vi "Example 5 - RMX410x Configuration.vi"(8 "error in (no error)":errorcluster) -> (0 "error out":errorcluster)   [LabVIEW 2018]
uses:
  <vilib>/addons/VeriStand Custom Device Scripting APIs/Instrument Addon/Libraries Directory/Protocols.lvlibp/RS-xxx/RS-xxx Settings.ctl
  <vilib>/addons/VeriStand Custom Device Scripting APIs/Instrument Addon/API/TypeDefs/Message Settings.ctl
  <vilib>/addons/VeriStand Custom Device Scripting APIs/Instrument Addon/API/TypeDefs/Protection Types.ctl
  <vilib>/addons/VeriStand Custom Device Scripting APIs/Instrument Addon/API/TypeDefs/Single Channel Enumerated List Settings.ctl
  <vilib>/NI Veristand/Custom Device API/Custom Device Item Ref.ctl
  <vilib>/addons/VeriStand Custom Device Scripting APIs/Instrument Addon/API/TypeDefs/Command Settings.ctl
  <vilib>/addons/VeriStand Custom Device Scripting APIs/Instrument Addon/API/TypeDefs/Padding.ctl
  <vilib>/addons/VeriStand Custom Device Scripting APIs/Instrument Addon/API/TypeDefs/ByteCount Response Settings.ctl
  <vilib>/addons/VeriStand Custom Device Scripting APIs/Instrument Addon/API/TypeDefs/Linked Channel.ctl
  <vilib>/addons/VeriStand Custom Device Scripting APIs/Instrument Addon/API/TypeDefs/Single Channel Format Settings.ctl
  NationalInstruments.VeriStand.SystemDefinitionAPI
  <vilib>/addons/VeriStand Custom Device Scripting APIs/Instrument Addon/API/Custom Device/RS-xxx Factory.vi
  <vilib>/addons/VeriStand Custom Device Scripting APIs/Instrument Addon/API/Messages/Create Message - Periodic & Trigger.vi
  <vilib>/addons/VeriStand Custom Device Scripting APIs/Instrument Addon/API/Channels/Create Data Channel - Single Channel - Format.vi
  <vilib>/addons/VeriStand Custom Device Scripting APIs/Instrument Addon/API/Messages/Configure Response - Byte Count.vi
  <vilib>/addons/VeriStand Custom Device Scripting APIs/Instrument Addon/API/Channels/Create Data Channel - Single Channel - Enumerated List.vi
  <vilib>/addons/VeriStand Custom Device Scripting APIs/Instrument Addon/API/Messages/Create Message - Value Change & Trigger.vi
  <vilib>/addons/VeriStand Custom Device Scripting APIs/Instrument Addon/API/Channels/Create MetaData Channel - Single Channel - Format.vi
  <vilib>/addons/VeriStand Custom Device Scripting APIs/Instrument Addon/API/Channels/Create MetaData Channel - Single Channel - Enumerated List.vi
  <vilib>/addons/VeriStand Custom Device Scripting APIs/Instrument Addon/API/Instrument Addon Scripting API.lvlib
  <vilib>/addons/VeriStand Custom Device Scripting APIs/Instrument Addon/Libraries Directory/Protocols.lvlibp/RS-xxx/RS-xxx.lvclass
  <vilib>/NI Veristand/Custom Device API/Custom Device API.lvlib
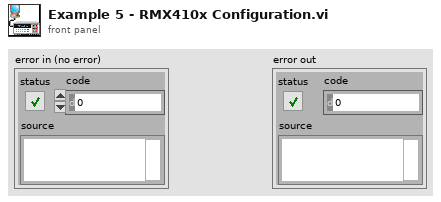
[diagram p1: front panel]
types:
  T1 = typedef "Instrument Addon Scripting API.lvlib/Linked Channel.ctl" = cluster{"Variable Name":string, "Channel Refnum":T2}
  T2 = typedef "Custom Device API.lvlib/Custom Device Item Ref.ctl" = u64
  T3 = typedef "Instrument Addon Scripting API.lvlib/ByteCount Response Settings.ctl" = cluster{"Response Format":string, "Linked Channels":T1[], "Byte Count":i32, "Use Byte Count channel":bool, "Channel Refnum":T2}
  T4 = typedef "Instrument Addon Scripting API.lvlib/Single Channel Format Settings.ctl" = cluster{"Format String":string, "Default Value":dbl, "Units":string}
  T5 = typedef "Instrument Addon Scripting API.lvlib/Single Channel Enumerated List Settings.ctl" = cluster{"Enumerated List":string[], "Default Value":dbl, "Units":string}
  T6 = cluster{"Variable Name":string, "Channel Ref in":T2}
  T7 = typedef "Instrument Addon Scripting API.lvlib/Command Settings.ctl" = cluster{"Command Format":string, "Linked Channels":cluster{"Variable Name":string, "Channel Ref in":T2}[], "Use Padding?":bool, "Padding":T8}
  T8 = typedef "Instrument Addon Scripting API.lvlib/Padding.ctl" = cluster{"Pad Value":u8, "Length":u32}
  T9 = typedef "Instrument Addon Scripting API.lvlib/Protection Types.ctl" = enum16{"None", "CRC-32", "Checksum U16", "Checksum U32", "Checksum U8"}
  T10 = typedef "Instrument Addon Scripting API.lvlib/Message Settings.ctl" = cluster{"Protection":T9, "Enable Periodic Default":bool, "Trigger Channel refnum":u64}
  T11 = enum16{"NUL", "SOH", "STX", "ETX", "EOT", "ENQ", "ACK", "BEL", "BS", "HT", "LF", "VT", "FF", "CR", "SO", "SI", "DLE", "DC1", "DC2", "DC3", "DC4", "NAK", "SYN", "ETB", "CAN", "EM", "SUB", "ESC", "FS", "GS", "RS", "US", "SP", "!", "\"", "#", "$", "%", "&", "'", "(", ")", "*", "+", ",", "- (-)", ".", "/", "0", "1", "2", "3", "4", "5", "6", "7", "8", "9", ":", ";", "<", "=", ">", "?", "@", "A", "B", "C", "D", "E", "F", "G", "H", "I", "J", "K", "L", "M", "N", "O", "P", "Q", "R", "S", "T", "U", "V", "W", "X", "Y", "Z", "[", "\\", "]", "^", "_", "`", "a", "b", "c", "d", "e", "f", "g", "h", "i", "j", "k", "l", "m", "n", "o", "p", "q", "r", "s", "t", "u", "v", "w", "x", "y", "z", "{", "|", "}", "~"}
  T12 = typedef "Protocols.lvlibp/RS-xxx.lvclass/RS-xxx Settings.ctl" = cluster{"Port":string, "Baud Rate":u32, "Data Bits":u16, "Parity":enum16{"None", "Odd", "Even", "Mark", "Space"}, "Stop Bits":u16, "Flow Control":u16, "XON":enum16{"NUL", "SOH", "STX", "ETX", "EOT", "ENQ", "ACK", "BEL", "BS", "HT", "LF", "VT", "FF", "CR", "SO", "SI", "DLE", "DC1", "DC2", "DC3", "DC4", "NAK", "SYN", "ETB", "CAN", "EM", "SUB", "ESC", "FS", "GS", "RS", "US", "SP", "!", "\"", "#", "$", "%", "&", "'", "(", ")", "*", "+", ",", "- (-)", ".", "/", "0", "1", "2", "3", "4", "5", "6", "7", "8", "9", ":", ";", "<", "=", ">", "?", "@", "A", "B", "C", "D", "E", "F", "G", "H", "I", "J", "K", "L", "M", "N", "O", "P", "Q", "R", "S", "T", "U", "V", "W", "X", "Y", "Z", "[", "\\", "]", "^", "_", "`", "a", "b", "c", "d", "e", "f", "g", "h", "i", "j", "k", "l", "m", "n", "o", "p", "q", "r", "s", "t", "u", "v", "w", "x", "y", "z", "{", "|", "}", "~"}, "XOFF":enum16{"NUL", "SOH", "STX", "ETX", "EOT", "ENQ", "ACK", "BEL", "BS", "HT", "LF", "VT", "FF", "CR", "SO", "SI", "DLE", "DC1", "DC2", "DC3", "DC4", "NAK", "SYN", "ETB", "CAN", "EM", "SUB", "ESC", "FS", "GS", "RS", "US", "SP", "!", "\"", "#", "$", "%", "&", "'", "(", ")", "*", "+", ",", "- (-)", ".", "/", "0", "1", "2", "3", "4", "5", "6", "7", "8", "9", ":", ";", "<", "=", ">", "?", "@", "A", "B", "C", "D", "E", "F", "G", "H", "I", "J", "K", "L", "M", "N", "O", "P", "Q", "R", "S", "T", "U", "V", "W", "X", "Y", "Z", "[", "\\", "]", "^", "_", "`", "a", "b", "c", "d", "e", "f", "g", "h", "i", "j", "k", "l", "m", "n", "o", "p", "q", "r", "s", "t", "u", "v", "w", "x", "y", "z", "{", "|", "}", "~"}, "End Read on Termination Character":bool, "End Write on Termination Character":bool, "Termination Character":u8}
  T13 = cluster{"Variable Name":string, "Channel Ref in":T2}[]
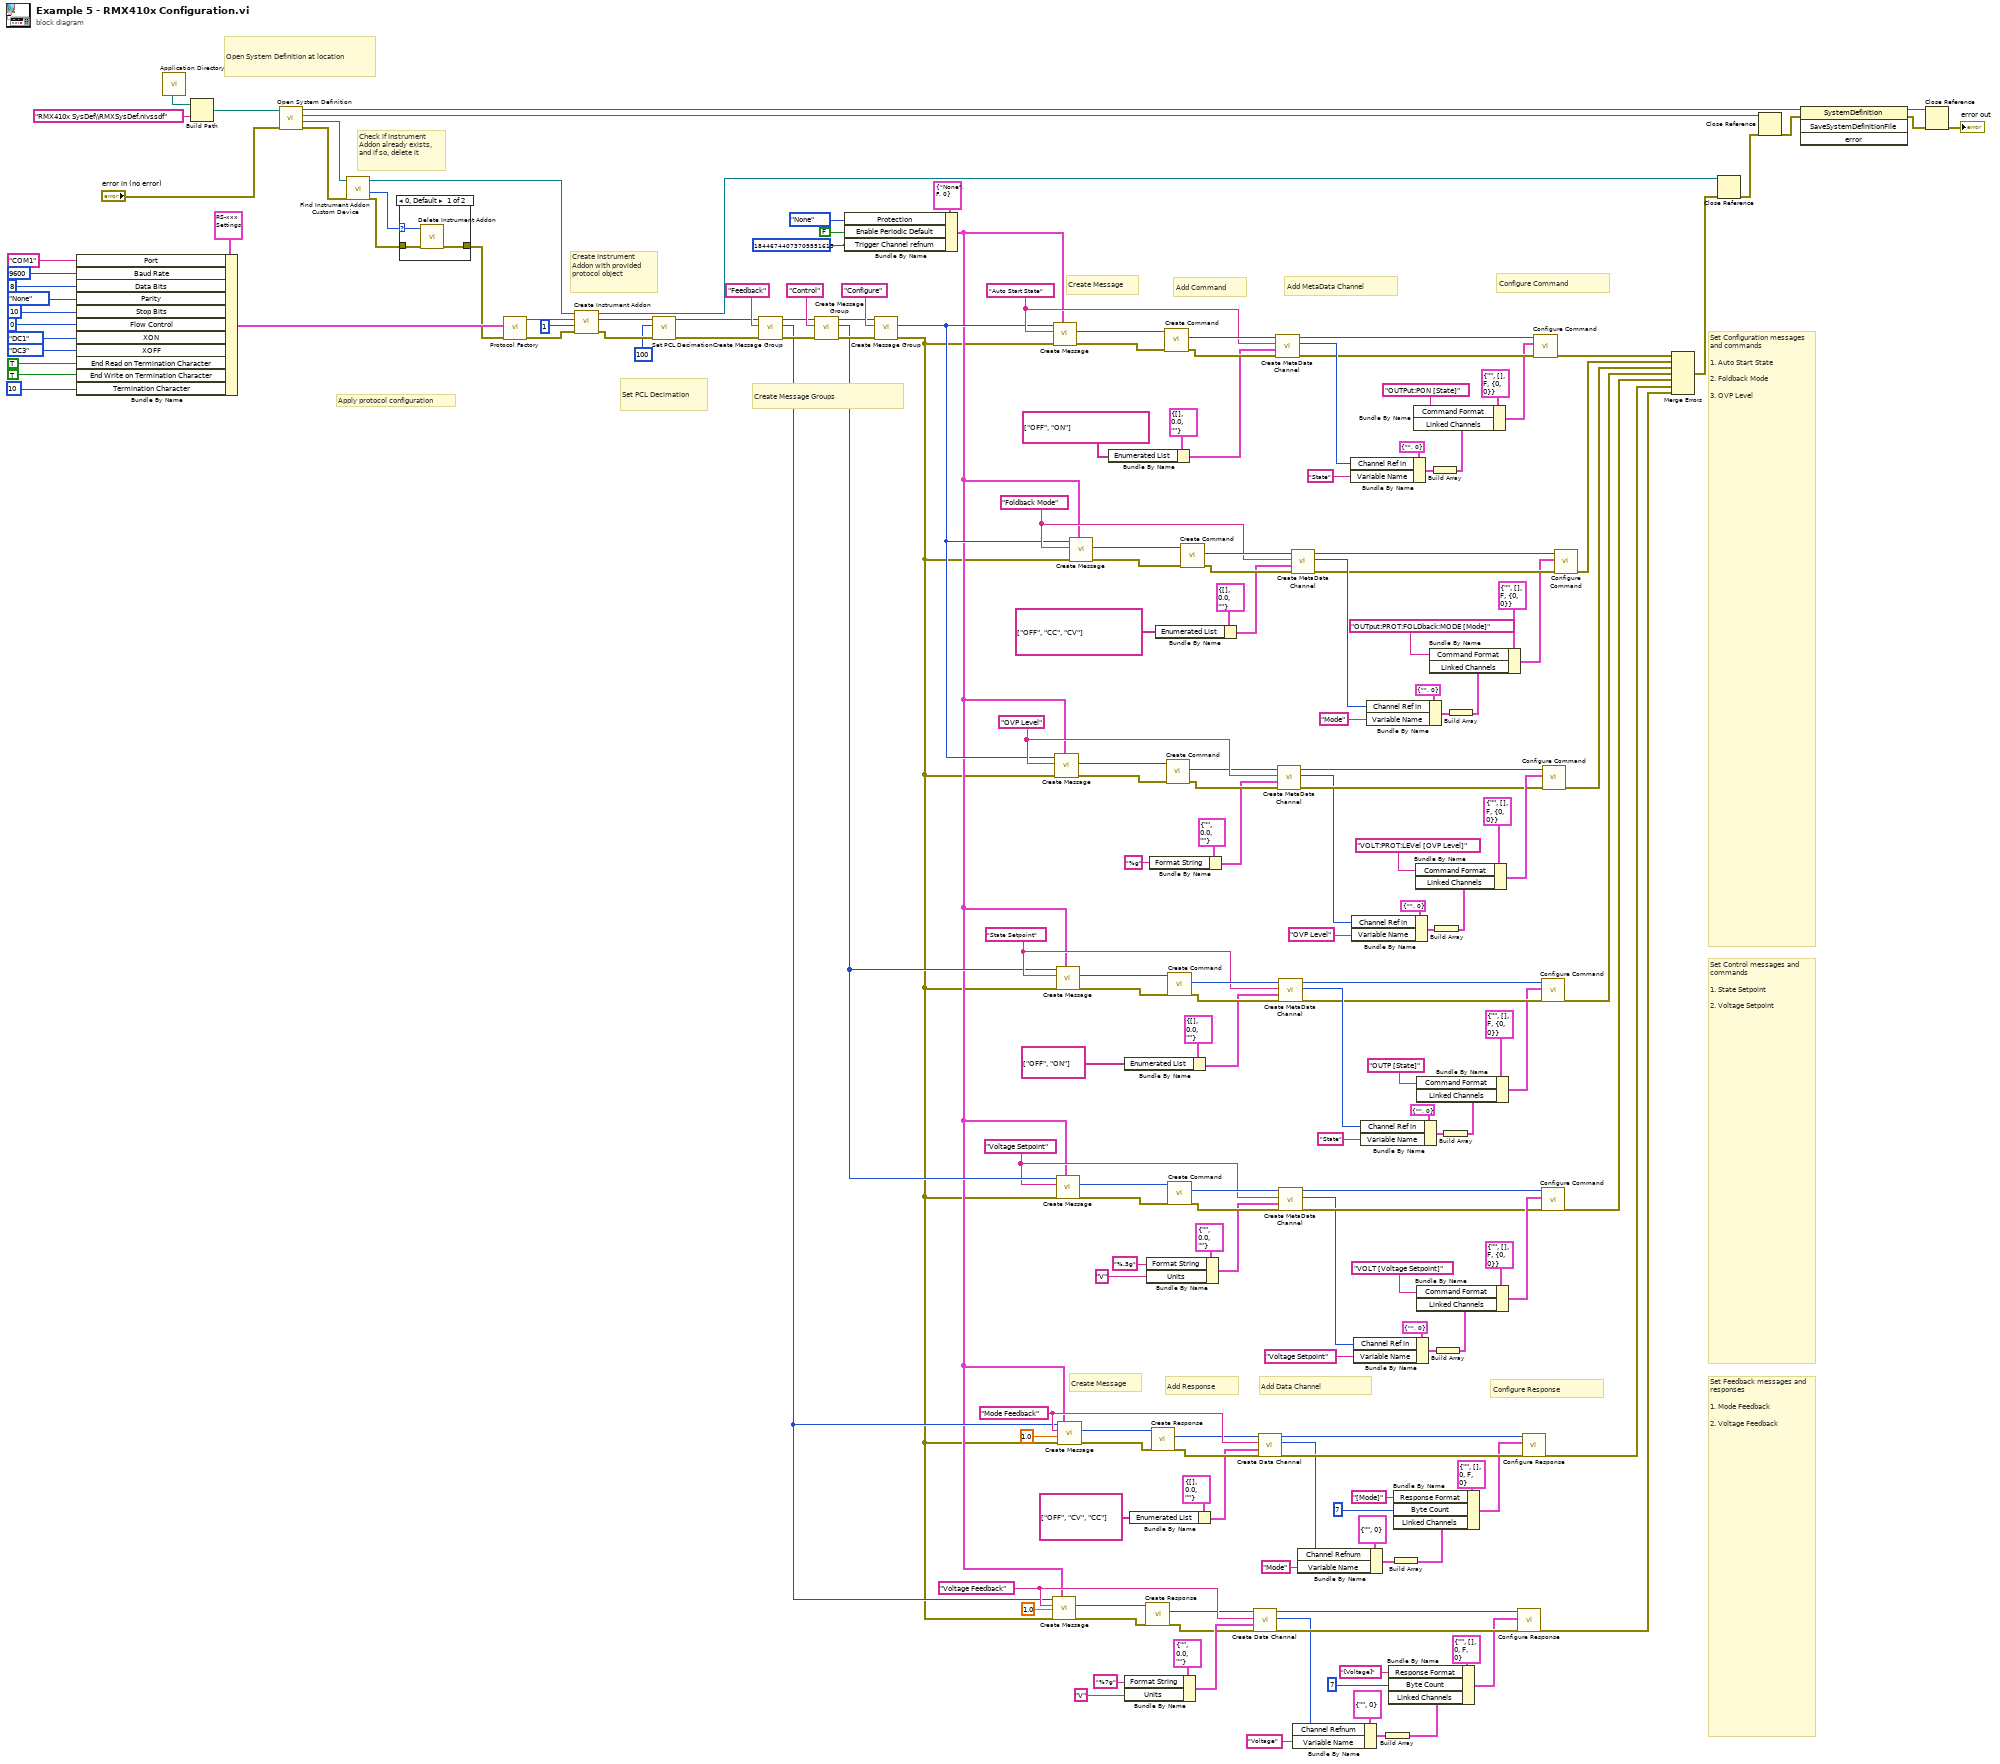
[diagram p0: block diagram]
diagram:
  w17 = "Voltage Feedback" ("message name")
  w40 = "Mode Feedback" ("message name")
  w58 = "Voltage Setpoint" ("message name")
  w78 = "State Setpoint" ("message name")
  w117 = "OVP Level" ("message name")
  w120 = "Foldback Mode" ("message name")
  w119 = "Auto Start State" ("message name")
  # "Create Instrument Addon with provided protocol object"
  # "Open System Definition at location"
  # "Configure Response"
  # "Add Data Channel"
  # "Add Response"
  # "Create Message"
  # "Configure Command"
  # "Add MetaData Channel"
  # "Add Command"
  # "Create Message"
  # "Set Feedback messages and responses\n\n1. Mode Feedback\n\n2. Voltage Feedback"
  # "Set Control messages and commands\n\n1. State Setpoint\n\n2. Voltage Setpoint"
  # "Set Configuration messages and commands\n\n1. Auto Start State\n\n2. Foldback Mode\n\n3. OVP Level"
  # "Create Message Groups"
  # "Set PCL Decimation"
  # "Check if Instrument Addon already exists, and if so, delete it"
  # "Apply protocol configuration"
  n1 = Bundle By Name(cluster=T12 {"Port"="", "Baud Rate"=0, "Data Bits"=0, "Parity"=enum."None", "Stop Bits"=0, "Flow Control"=0, "XON"=enum."NUL", "XOFF"=enum."NUL", "End Read on Termination Character"=FALSE, "End Write on Termination Character"=FALSE, "Termination Character"=0} ("RS-xxx settings"), "Port"="COM1", "Baud Rate"=u32 9600, "Data Bits"=u16 8, "Parity"=enum16{"None", "Odd", "Even", "Mark", "Space"}."None", "Stop Bits"=u16 10, "Flow Control"=u16 0, "XON"=T11."DC1", "XOFF"=T11."DC3", "End Read on Termination Character"=TRUE, "End Write on Termination Character"=TRUE ("End Read on Termination Character"), "Termination Character"=u8 10) -> (w193:T12)
  n2 = call <vilib>:"Application Directory.vi"() -> ("Application Directory"=w180:path)
  n3 = Build Path(base path=w180, name or relative path="RMX410x SysDef\\RMXSysDef.nivssdf") -> (appended path=w178:path)
  n4 = call "Open System Definition.vi"("error in (no error)"="error in (no error)", "System Definition File"=w178) -> ("error out"=w166:errorcluster, "Target Refnum"=w168:refnum<k24>, "Root Refnum"=w177:refnum<k24>, "System Definition Refnum"=w172:refnum<k24>)  [unwired: 6 in]
  n5 = call "Find Instrument Addon Custom Device.vi"("error in"=w166, "target in"=w168) -> ("error out"=w165:errorcluster, "NodeID"=w147:u64, "target out"=w163:refnum<k24>)  [unwired: 7 in]
  n6 = case shown="0, Default" w147 {
    selector: w147 -> [w196 _]
    tunnel: w165 -> [w198 w199]
    tunnel: [w197 w199] -> w164
    frame 0, Default {
      n7 = call <vilib>:"Delete Instrument Addon.vi"("error in (no error)"=w198, "instrument addon refnum"=w196) -> ("error out"=w197:errorcluster)  [unwired: 9 in]
    }
    frame -1 {
    }
  }
  n8 = call-poly <vilib>:"Protocol Factory.vi"("error in (no error)"=w164, "RS-xxx settings"=w193) -> ("error out"=w175:errorcluster, "protocol out"=w195:refnum<class "Protocol Parent.lvclass">)  [unwired: 8 in]
  n9 = call <vilib>:"Create Instrument Addon.vi"("error in (no error)"=w175, "PCL decimation"=u16 1, "protocol in"=w195, "target in"=w163) -> ("error out"=w8:errorcluster, "instrument addon refnum"=w9:T2, "target out"=w176:refnum<k24>)  [unwired: 5 in]
  n10 = call <vilib>:"Set PCL Decimation.vi"("error in (no error)"=w8, "PCL decimation"=u32 100, "instrument addon refnum in"=w9) -> ("error out"=w6:errorcluster, "instrument addon refnum"=w7:T2)  [unwired: 7 in]
  n11 = call <vilib>:"Create Message Group.vi"("error in (no error)"=w6, "message group name"="Feedback", "instrument addon refnum in"=w7) -> ("error out"=w95:errorcluster, "message group refnum out"=w12:T2, "instrument addon refnum out"=w96:T2)  [unwired: 6 in]
  n12 = call <vilib>:"Create Message Group.vi"("error in (no error)"=w95, "message group name"="Control", "instrument addon refnum in"=w96) -> ("error out"=w93:errorcluster, "message group refnum out"=w59:T2, "instrument addon refnum out"=w94:T2)  [unwired: 6 in]
  n13 = Bundle By Name(cluster=T10 {"Protection"=enum."None", "Enable Periodic Default"=FALSE, "Trigger Channel refnum"=0} ("optional settings"), "Protection"=Protection_Types."None", "Enable Periodic Default"=FALSE, "Trigger Channel refnum"=T2 18446744073709551615 ("command refnum")) -> (w4:T10)
  n14 = call <vilib>:"Create Message Group.vi"("error in (no error)"=w93, "message group name"="Configure", "instrument addon refnum in"=w94) -> ("error out"=w3:errorcluster, "message group refnum out"=w74:T2)  [unwired: 6 in, 1 out]
  n15 = call-poly <vilib>:"Create Message.vi"("optional settings"=w4, "error in (no error)"=w3, "period (s)"=1.0, "message name"=w17, "message group refnum in"=w12) -> ("error out"=w14:errorcluster, "message refnum out"=w13:T2)  [unwired: 4 in, 1 out]
  n16 = call-poly <vilib>:"Create Message.vi"("optional settings"=w4, "error in (no error)"=w3, "message name"=w119, "message group refnum in"=w74) -> ("error out"=w160:errorcluster, "message refnum out"=w161:T2)  [unwired: 5 in, 1 out]
  n17 = call-poly <vilib>:"Create Message.vi"("optional settings"=w4, "error in (no error)"=w3, "message name"=w117, "message group refnum in"=w74) -> ("error out"=w104:errorcluster, "message refnum out"=w103:T2)  [unwired: 5 in, 1 out]
  n18 = call-poly <vilib>:"Create Message.vi"("optional settings"=w4, "error in (no error)"=w3, "message name"=w78, "message group refnum in"=w59) -> ("error out"=w91:errorcluster, "message refnum out"=w92:T2)  [unwired: 5 in, 1 out]
  n19 = call-poly <vilib>:"Create Message.vi"("optional settings"=w4, "error in (no error)"=w3, "message name"=w58, "message group refnum in"=w59) -> ("error out"=w61:errorcluster, "message refnum out"=w60:T2)  [unwired: 5 in, 1 out]
  n20 = call-poly <vilib>:"Create Message.vi"("optional settings"=w4, "error in (no error)"=w3, "period (s)"=1.0, "message name"=w40, "message group refnum in"=w12) -> ("error out"=w37:errorcluster, "message refnum out"=w36:T2)  [unwired: 4 in, 1 out]
  n21 = call-poly <vilib>:"Create Message.vi"("optional settings"=w4, "error in (no error)"=w3, "message name"=w120, "message group refnum in"=w74) -> ("error out"=w136:errorcluster, "message refnum out"=w137:T2)  [unwired: 5 in, 1 out]
  n22 = Bundle By Name(cluster=T5 {"Enumerated List"=[], "Default Value"=0.0, "Units"=""} ("settings"), "Enumerated List"=string[] ["OFF", "ON"]) -> (w155:T5)
  n23 = Bundle By Name(cluster=T5 {"Enumerated List"=[], "Default Value"=0.0, "Units"=""} ("settings"), "Enumerated List"=string[] ["OFF", "ON"]) -> (w76:T5)
  n24 = Bundle By Name(cluster=T4 {"Format String"="", "Default Value"=0.0, "Units"=""} ("settings"), "Format String"="%7g", "Units"="V") -> (w19:T4)
  n25 = Bundle By Name(cluster=T5 {"Enumerated List"=[], "Default Value"=0.0, "Units"=""} ("settings"), "Enumerated List"=string[] ["OFF", "CV", "CC"]) -> (w34:T5)
  n26 = call <vilib>:"Create Response.vi"("error in (no error)"=w14, "message refnum in"=w13) -> ("error out"=w16:errorcluster, "response refnum"=w15:T2)  [unwired: 7 in, 1 out]
  n27 = Bundle By Name(cluster=T4 {"Format String"="", "Default Value"=0.0, "Units"=""} ("settings"), "Format String"="%.3g", "Units"="V") -> (w56:T4)
  n28 = Bundle By Name(cluster=T4 {"Format String"="", "Default Value"=0.0, "Units"=""} ("settings"), "Format String"="%g") -> (w101:T4)
  n29 = call <vilib>:"Create Response.vi"("error in (no error)"=w37, "message refnum in"=w36) -> ("error out"=w39:errorcluster, "response refnum"=w38:T2)  [unwired: 7 in, 1 out]
  n30 = Bundle By Name(cluster=T5 {"Enumerated List"=[], "Default Value"=0.0, "Units"=""} ("settings"), "Enumerated List"=string[] ["OFF", "CC", "CV"]) -> (w131:T5)
  n31 = call <vilib>:"Create Command.vi"("error in"=w160, "message refnum In"=w161) -> ("error out"=w158:errorcluster, "command refnum"=w159:T2)  [unwired: 7 in, 1 out]
  n32 = call <vilib>:"Create Command.vi"("error in"=w104, "message refnum In"=w103) -> ("error out"=w106:errorcluster, "command refnum"=w105:T2)  [unwired: 7 in, 1 out]
  n33 = call <vilib>:"Create Command.vi"("error in"=w91, "message refnum In"=w92) -> ("error out"=w89:errorcluster, "command refnum"=w90:T2)  [unwired: 7 in, 1 out]
  n34 = call <vilib>:"Create Command.vi"("error in"=w61, "message refnum In"=w60) -> ("error out"=w63:errorcluster, "command refnum"=w62:T2)  [unwired: 7 in, 1 out]
  n35 = call <vilib>:"Create Command.vi"("error in"=w136, "message refnum In"=w137) -> ("error out"=w134:errorcluster, "command refnum"=w135:T2)  [unwired: 7 in, 1 out]
  n36 = call-poly <vilib>:"Create Data Channel.vi"("error in (no error)"=w16, "settings"=w19, "channel name"=w17, "response refnum in"=w15) -> ("error out"=w32:errorcluster, "channel refnum"=w27:T2, "response refnum out"=w22:T2)  [unwired: 5 in]
  n37 = call-poly <vilib>:"Create Data Channel.vi"("error in (no error)"=w39, "settings"=w34, "channel name"=w40, "response refnum in"=w38) -> ("error out"=w51:errorcluster, "channel refnum"=w46:T2, "response refnum out"=w41:T2)  [unwired: 5 in]
  n38 = call-poly <vilib>:"Create MetaData Channel.vi"("error in (no error)"=w158, "settings"=w155, "channel name"=w119, "command refnum in"=w159) -> ("error out"=w152:errorcluster, "channel refnum"=w153:T2, "command refnum out"=w154:T2)  [unwired: 5 in]
  n39 = call-poly <vilib>:"Create MetaData Channel.vi"("error in (no error)"=w106, "settings"=w101, "channel name"=w117, "command refnum in"=w105) -> ("error out"=w109:errorcluster, "channel refnum"=w108:T2, "command refnum out"=w107:T2)  [unwired: 5 in]
  n40 = call-poly <vilib>:"Create MetaData Channel.vi"("error in (no error)"=w89, "settings"=w76, "channel name"=w78, "command refnum in"=w90) -> ("error out"=w86:errorcluster, "channel refnum"=w87:T2, "command refnum out"=w88:T2)  [unwired: 5 in]
  n41 = call-poly <vilib>:"Create MetaData Channel.vi"("error in (no error)"=w63, "settings"=w56, "channel name"=w58, "command refnum in"=w62) -> ("error out"=w66:errorcluster, "channel refnum"=w65:T2, "command refnum out"=w64:T2)  [unwired: 5 in]
  n42 = call-poly <vilib>:"Create MetaData Channel.vi"("error in (no error)"=w134, "settings"=w131, "channel name"=w120, "command refnum in"=w135) -> ("error out"=w128:errorcluster, "channel refnum"=w129:T2, "command refnum out"=w130:T2)  [unwired: 5 in]
  n43 = Bundle By Name(cluster=T1 {"Variable Name"="", "Channel Refnum"=0} ("Linked Channel"), "Channel Refnum"=w27, "Variable Name"="Voltage") -> (w29:T1)
  n44 = Bundle By Name(cluster=T1 {"Variable Name"="", "Channel Refnum"=0} ("Linked Channel"), "Channel Refnum"=w46, "Variable Name"="Mode") -> (w48:T1)
  n45 = Bundle By Name(cluster=T6 {"Variable Name"="", "Channel Ref in"=0} ("Linked Channel"), "Channel Ref in"=w153, "Variable Name"="State") -> (w142:T6)
  n46 = Bundle By Name(cluster=T6 {"Variable Name"="", "Channel Ref in"=0} ("Linked Channel"), "Channel Ref in"=w108, "Variable Name"="OVP Level") -> (w114:T6)
  n47 = Bundle By Name(cluster=T6 {"Variable Name"="", "Channel Ref in"=0} ("Linked Channel"), "Channel Ref in"=w65, "Variable Name"="Voltage Setpoint") -> (w71:T6)
  n48 = Bundle By Name(cluster=T6 {"Variable Name"="", "Channel Ref in"=0} ("Linked Channel"), "Channel Ref in"=w87, "Variable Name"="State") -> (w81:T6)
  n49 = Bundle By Name(cluster=T6 {"Variable Name"="", "Channel Ref in"=0} ("Linked Channel"), "Channel Ref in"=w129, "Variable Name"="Mode") -> (w123:T6)
  n50 = Build Array(w29) -> (w30:T1[])
  n51 = Bundle By Name(cluster=T3 {"Response Format"="", "Linked Channels"=[], "Byte Count"=0, "Use Byte Count channel"=FALSE, "Channel Refnum"=0} ("settings"), "Response Format"="[Voltage]", "Byte Count"=7, "Linked Channels"=w30) -> (w25:T3)
  n52 = Build Array(w48) -> (w49:T1[])
  n53 = Bundle By Name(cluster=T3 {"Response Format"="", "Linked Channels"=[], "Byte Count"=0, "Use Byte Count channel"=FALSE, "Channel Refnum"=0} ("settings"), "Response Format"="[Mode]", "Byte Count"=7, "Linked Channels"=w49) -> (w44:T3)
  n54 = Build Array(w142) -> (w141:T13)
  n55 = Bundle By Name(cluster=T7 {"Command Format"="", "Linked Channels"=[], "Use Padding?"=FALSE, "Padding"={"Pad Value"=0, "Length"=0}} ("settings"), "Command Format"="OUTPut:PON [State]", "Linked Channels"=w141) -> (w140:T7)
  n56 = Build Array(w114) -> (w115:T13)
  n57 = Bundle By Name(cluster=T7 {"Command Format"="", "Linked Channels"=[], "Use Padding?"=FALSE, "Padding"={"Pad Value"=0, "Length"=0}} ("settings"), "Command Format"="VOLT:PROT:LEVel [OVP Level]", "Linked Channels"=w115) -> (w116:T7)
  n58 = Build Array(w71) -> (w72:T13)
  n59 = Bundle By Name(cluster=T7 {"Command Format"="", "Linked Channels"=[], "Use Padding?"=FALSE, "Padding"={"Pad Value"=0, "Length"=0}} ("settings"), "Command Format"="VOLT [Voltage Setpoint]", "Linked Channels"=w72) -> (w73:T7)
  n60 = Build Array(w81) -> (w80:T13)
  n61 = Bundle By Name(cluster=T7 {"Command Format"="", "Linked Channels"=[], "Use Padding?"=FALSE, "Padding"={"Pad Value"=0, "Length"=0}} ("settings"), "Command Format"="OUTP [State]", "Linked Channels"=w80) -> (w79:T7)
  n62 = Build Array(w123) -> (w122:T13)
  n63 = Bundle By Name(cluster=T7 {"Command Format"="", "Linked Channels"=[], "Use Padding?"=FALSE, "Padding"={"Pad Value"=0, "Length"=0}} ("settings"), "Command Format"="OUTput:PROT:FOLDback:MODE [Mode]", "Linked Channels"=w122) -> (w121:T7)
  n64 = call-poly <vilib>:"Configure Response.vi"("error in (no error)"=w32, "settings"=w25, "response refnum in"=w22) -> ("error out"=w11:errorcluster)  [unwired: 7 in, 1 out]
  n65 = call-poly <vilib>:"Configure Response.vi"("error in (no error)"=w51, "settings"=w44, "response refnum in"=w41) -> ("error out"=w10:errorcluster)  [unwired: 7 in, 1 out]
  n66 = call <vilib>:"Configure Command.vi"("error in (no error)"=w152, "settings"=w140, "command refnum in"=w154) -> ("error out"=w139:errorcluster)  [unwired: 7 in, 1 out]
  n67 = call <vilib>:"Configure Command.vi"("error in (no error)"=w86, "settings"=w79, "command refnum in"=w88) -> ("error out"=w54:errorcluster)  [unwired: 7 in, 1 out]
  n68 = call <vilib>:"Configure Command.vi"("error in (no error)"=w66, "settings"=w73, "command refnum in"=w64) -> ("error out"=w52:errorcluster)  [unwired: 7 in, 1 out]
  n69 = call <vilib>:"Configure Command.vi"("error in (no error)"=w109, "settings"=w116, "command refnum in"=w107) -> ("error out"=w99:errorcluster)  [unwired: 7 in, 1 out]
  n70 = call <vilib>:"Configure Command.vi"("error in (no error)"=w128, "settings"=w121, "command refnum in"=w130) -> ("error out"=w118:errorcluster)  [unwired: 7 in, 1 out]
  n71 = Merge Errors(w139, w118, w99, w54, w52, w10, w11) -> (w138:errorcluster)
  n72 = Close Reference(reference=w176, error in (no error)=w138) -> (error out=w174:errorcluster)
  n73 = Close Reference(reference=w177, error in (no error)=w174) -> (error out=w171:errorcluster)
  n74 = invoke class="SystemDefinition" method="SaveSystemDefinitionFile"(reference=w172, error in=w171) -> (reference out=w170:refnum<k24>, error out=w169:errorcluster)  [unwired: 2 in, 2 out]
  n75 = Close Reference(reference=w170, error in (no error)=w169) -> (error out=→"error out":errorcluster)
